vi "Flatten Value.vi"(8 "error in (no error)":errorcluster, 11 "Boolean in":refnum<class "Assertion.lvclass">) -> (0 "error out":errorcluster, 2 "Value":string, 3 "Boolean out":refnum<class "Assertion.lvclass">)   [LabVIEW 2019, in "Assertion.lvclass"]
uses:
  <vilib>/gpm_packages/@cs/data-type-serializer/source/Assertion/Assertion.lvclass
  <vilib>/gpm_packages/@cs/data-type-serializer/source/Assertion/Assertion.lvclass/Assertion.ctl
  <vilib>/gpm_packages/@cs/run-time-assertions/Source/Assert/Assert.lvclass
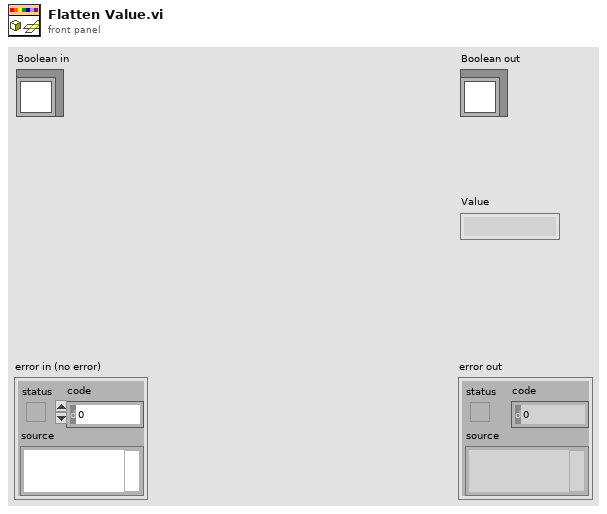
[diagram p1: front panel]
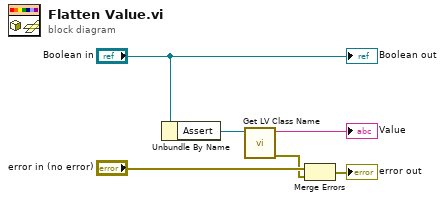
[diagram p0: block diagram]
diagram:
  n1 = Unbundle By Name("Boolean in") -> ("Assert"=w3:refnum<class "Assert.lvclass">)
  n2 = call <vilib>:"Get LV Class Name.vi"("object"=w3) -> ("error out"=w2:errorcluster, "class name"=→"Value":string)  [unwired: 9 in]
  n3 = Merge Errors("error in (no error)", w2) -> (→"error out":errorcluster)
  "Boolean out" <- "Boolean in"
